vi "Set Jog High Speed.vi"(4 "error in (no error)":errorcluster, 5 "Jog High Speed (0 units/s)":dbl min=0.0 format="%.6g", 6 "Axis (1)":i32=1 min=1 max=3, 7 "VISA resource name":refnum<visa-resource-name>) -> (0 "error out":errorcluster, 3 "VISA resource name out":refnum<visa-resource-name>)   [LabVIEW 2010, in "Newport ESP301.lvlib"]
doc: "This command is used to set the high speed for jogging an axis. Its execution is immediate, meaning that the value is changed when the command is processed, including when motion is in progress. It can be used as an immediate command or inside a program."
uses:
  <userlib>/Newport ESP301/Newport ESP301.lvlib
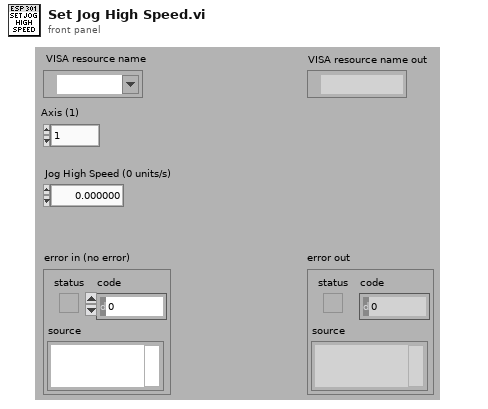
[diagram p1: front panel]
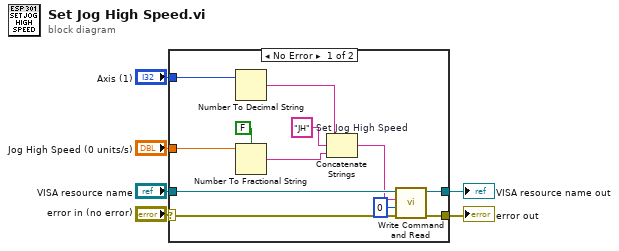
[diagram p0: block diagram]
diagram:
  n1 = case shown="No Error" "error in (no error)" {
    selector: "error in (no error)" -> [w15 w20]
    tunnel: [w17 w20] -> w6
    tunnel: "VISA resource name" -> [w18 w19]
    tunnel: [w16 w19] -> w5
    tunnel: "Jog High Speed (0 units/s)" -> [w14 _]
    tunnel: "Axis (1)" -> [w13 _]
    frame No Error {
      w12 = "JH"  # Set Jog High Speed
      n2 = Number To Decimal String(number=w13) -> (decimal integer string=w11:string)  [unwired: 1 in]
      n3 = Number To Fractional String(use system decimal point (T)=FALSE ("utiliser le séparateur décimal du système (V)"), number=w14) -> (F-format string=w10:string)  [unwired: 2 in]
      n4 = Concatenate Strings(w11, w12, w10) -> (w9:string)
      n5 = call <userlib>:"Write Command and Read.vi"("error in (no error)"=w15, "Bytes to read (100)"=u32 0, "Command"=w9, "VISA resource name"=w18) -> ("error out"=w17:errorcluster, "VISA resource name out"=w16:refnum<visa-resource-name>)  [unwired: 3 in, 1 out]
    }
    frame Error {
    }
  }
  "error out" <- w6
  "VISA resource name out" <- w5
